vi "CONFIG SPARK MAX PIDF.vi"(0 "MotorControlDevRef":T3, 2 "MOTOR PIDF coefficients":T1={"PIDF"={"P Gain"=0.001, "I Gain"=0.0, "D Gain"=0.0, "F Gain"=0.0012, "I Zone"=0.0, "Min Output"=-1.0, "Max Output"=1.0}, "Smart Motion"={"Max Velocity"=1900.0, "Max Acceleration"=750.0, "Minimum Velocity Output"=0.1, "Allowed Closed Loop Error"=0.02}}, 5 "error in (no error)":errorcluster, 9 "PIDF Slot":i32) -> (14 "MotorControlDevRef OUT":T3, 19 "error out":errorcluster)   [LabVIEW 2023]
uses:
  <vilib>/Rock Robotics/WPI/ThirdParty/REV Robotics/REVLib/SubVI/Public/SPARK Configure Closed Loop Smart Motion.vi
  <vilib>/Rock Robotics/WPI/ThirdParty/REV Robotics/REVLib/SubVI/Public/SPARK Configure Closed Loop Gains.vi
  <vilib>/Rock Robotics/WPI/ThirdParty/REV Robotics/REVLib/Typedef/SPARK Closed Loop Slot.ctl
  <vilib>/Rock Robotics/WPI/ThirdParty/REV Robotics/REVLib/Typedef/SPARK PID Gains.ctl
  <vilib>/Rock Robotics/WPI/ThirdParty/REV Robotics/REVLib/Typedef/SPARK Feed Forward Gains.ctl
  <vilib>/Rock Robotics/WPI/ThirdParty/REV Robotics/REVLib/Typedef/Spark MAX Smart Motion Parameters.ctl
  <vilib>/Rock Robotics/SystemInterfaces/DIO/FPGA_DIOPWMChannel.ctl
  <vilib>/Rock Robotics/WPI/PWM/WPI_PWMDeadband.ctl
  <vilib>/Rock Robotics/WPI/MotorControl/WPI_MotorControlType.ctl
  <vilib>/Rock Robotics/SystemInterfaces/DIO/FPGA_DIOChannel.ctl
  <vilib>/Rock Robotics/WPI/MotorControl/WPI_MotorControlDeviceRef.ctl
  ctrl defs/ctrl motor PIDF coefficients.ctl
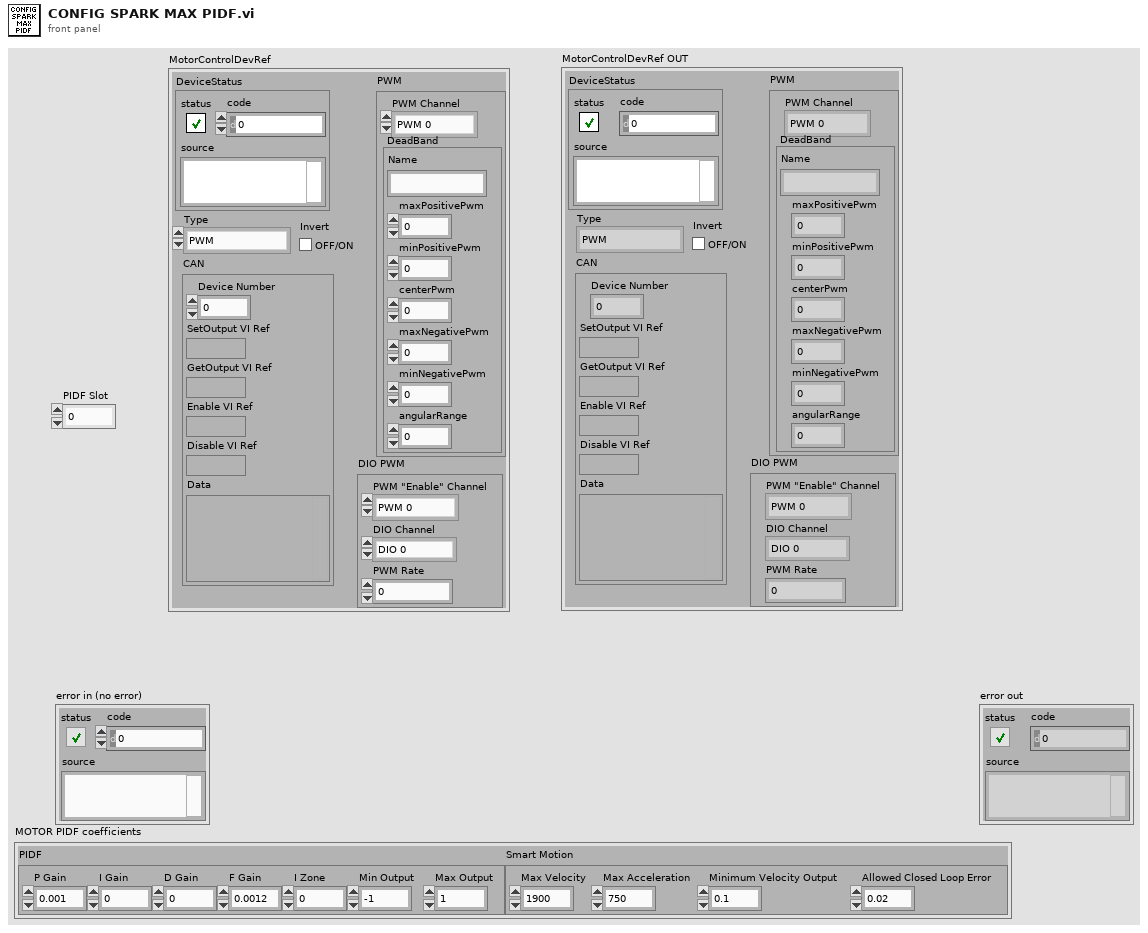
[diagram p1: front panel]
types:
  T1 = typedef "ctrl motor PIDF coefficients.ctl" = cluster{"PIDF":cluster{"P Gain":dbl, "I Gain":dbl, "D Gain":dbl, "F Gain":dbl, "I Zone":dbl, "Min Output":dbl, "Max Output":dbl}, "Smart Motion":T2}
  T2 = typedef "Spark MAX Smart Motion Parameters.ctl" = cluster{"Max Velocity":dbl, "Max Acceleration":dbl, "Minimum Velocity Output":dbl, "Allowed Closed Loop Error":dbl}
  T3 = typedef "WPI_MotorControlDeviceRef.ctl" = cluster{"DeviceStatus":errorcluster, "Type":T4, "PWM":cluster{"PWM Channel":T5, "DeadBand":T6}, "CAN":cluster{"Device Number":u8, "SetOutput VI Ref":variant, "GetOutput VI Ref":variant, "Enable VI Ref":variant, "Disable VI Ref":variant, "Data":variant}, "Invert":bool, "DIO PWM":cluster{"PWM \"Enable\" Channel":T5, "DIOChannel":T7, "PWM Rate":dbl}}
  T4 = typedef "WPI_MotorControlType.ctl" = enum16{"PWM", "CAN", "DIO PWM"}
  T5 = typedef "FPGA_DIOPWMChannel.ctl" = enum8{"PWM 0", "PWM 1", "PWM 2", "PWM 3", "PWM 4", "PWM 5", "PWM 6", "PWM 7", "PWM 8", "PWM 9", "PWM MXP 0", "PWM MXP 1", "PWM MXP 2", "PWM MXP 3", "PWM MXP 4", "PWM MXP 5", "PWM MXP 6", "PWM MXP 7", "PWM MXP 8", "PWM MXP 9", "Invalid"}
  T6 = typedef "WPI_PWMDeadband.ctl" = cluster{"Name":string, "maxPositivePwm":i32, "minPositivePwm":i32, "centerPwm":i32, "maxNegativePwm":i32, "minNegativePwm":i32, "angularRange":u16}
  T7 = typedef "FPGA_DIOChannel.ctl" = enum8{"DIO 0", "DIO 1", "DIO 2", "DIO 3", "DIO 4", "DIO 5", "DIO 6", "DIO 7", "DIO 8", "DIO 9", "DIO MXP 0", "DIO MXP 1", "DIO MXP 2", "DIO MXP 3", "DIO MXP 4", "DIO MXP 5", "DIO MXP 6", "DIO MXP 7", "DIO MXP 8", "DIO MXP 9", "DIO MXP 10", "DIO MXP 11", "DIO MXP 12", "DIO MXP 13", "DIO MXP 14", "DIO MXP 15", "SPI Port CS1", "SPI Port CS2", "SPI Port CS3", "SPI Port MISO", "SPI Port MOSI", "Invalid"}
  T8 = typedef "SPARK Feed Forward Gains.ctl" = cluster{"kV":dbl}
  T9 = typedef "SPARK PID Gains.ctl" = cluster{"kP":dbl, "kI":dbl, "kD":dbl}
  T10 = typedef "SPARK Closed Loop Slot.ctl" = u16
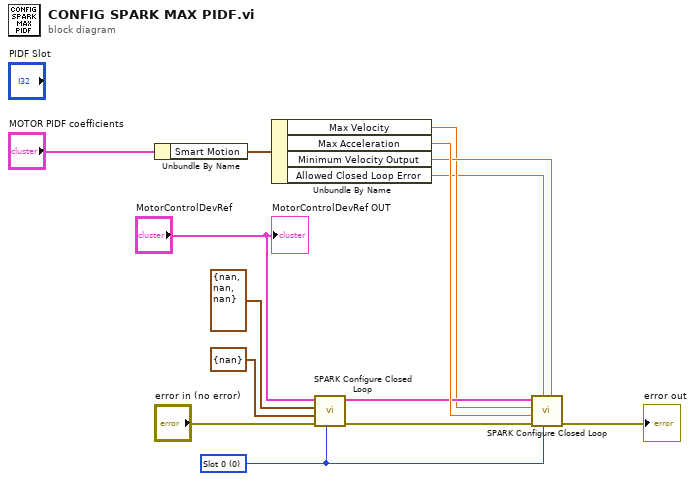
[diagram p0: block diagram]
diagram:
  w3 = T10 0 items=["Slot 0", "Slot 1", "Slot 2", "Slot 3"] ("Closed Loop Slot (0)")
  n1 = Unbundle By Name("MOTOR PIDF coefficients") -> ("Smart Motion"=w7:T2)
  n2 = Unbundle By Name(w7) -> ("Max Velocity"=w5:dbl, "Max Acceleration"=w14:dbl, "Minimum Velocity Output"=w6:dbl, "Allowed Closed Loop Error"=w4:dbl)
  n3 = call-poly <vilib>:"SPARK Configure Closed Loop.vi"("Closed Loop Slot (0)"=w3, "error in"="error in (no error)", "Feed Forward Gains"=T8 {"kV"=nan}, "PID Gains"=T9 {"kP"=nan, "kI"=nan, "kD"=nan}, "MotorControlDeviceRef in"="MotorControlDevRef") -> ("error out"=w12:errorcluster, "MotorControlDeviceRef out"=w11:T3)  [unwired: 5 in]
  n4 = call-poly <vilib>:"SPARK Configure Closed Loop.vi"("Min Velocity Output"=w6, "Closed Loop Slot (0)"=w3, "Allowed Closed Loop Error"=w4, "error in"=w12, "Max Acceleration"=w14, "Max Velocity"=w5, "MotorControlDeviceRef in"=w11) -> ("error out"=→"error out":errorcluster)  [unwired: 3 in, 1 out]
  "MotorControlDevRef OUT" <- "MotorControlDevRef"
